vi "hashString.vi"(8 "error in (no error)":errorcluster, 10 "String":string, 11 "HashMap in":refnum<class "HashMap.lvclass">) -> (0 "error out":errorcluster, 2 "Hash":i32, 3 "HashMap out":refnum<class "HashMap.lvclass">)   [LabVIEW 2017, in "HashMap.lvclass"]
uses:
  <userlib>/836-Library/Data_Structures/HashMap/HashMap.lvclass
  <userlib>/836-Library/Data_Structures/HashMap/HashMap.lvclass/HashMap.ctl
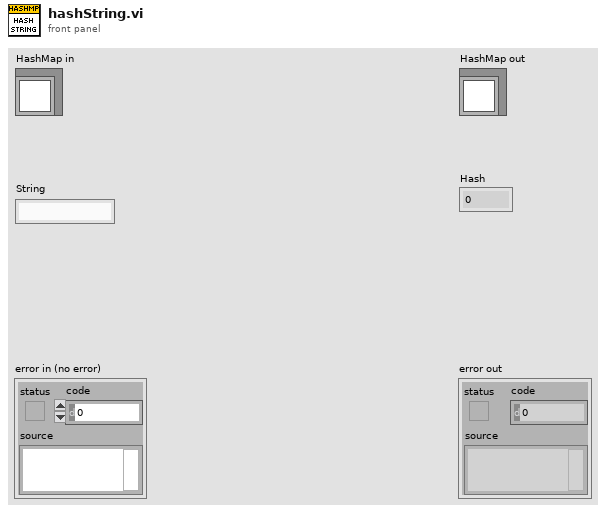
[diagram p1: front panel]
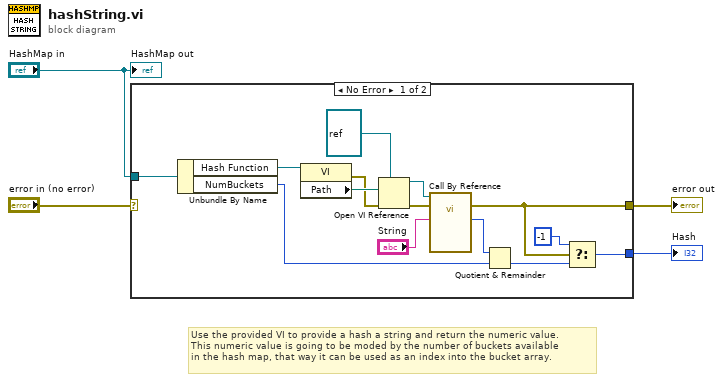
[diagram p0: block diagram]
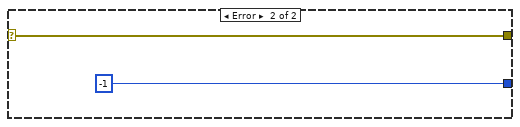
[diagram p2: hidden frame]
diagram:
  # "Use the provided VI to provide a hash a string and return the numeric value.\nThis numeric value is going to be moded by the number of buckets available\nin the hash map, that way it can be used as an index into the bucket array."
  n1 = case shown="No Error" "error in (no error)" {
    selector: "error in (no error)" -> [_ w20]
    tunnel: [w8 w20] -> w3
    tunnel: "HashMap in" -> [w18 _]
    tunnel: [w7 -1] -> w1
    frame No Error {
      n2 = Unbundle By Name(w18) -> ("Hash Function"=w17:refnum<vi>, "NumBuckets"=w9:i32)
      n3 = property class="VI"(reference=w17) -> (error out=w15:errorcluster, "Path"=w16:path)  [unwired: 1 in, 1 out]
      n4 = Open VI Reference(type specifier VI Refnum (for type only)=refnum<vi> refnum, vi path=w16, error in (no error)=w15) -> (vi reference=w13:refnum<vi>, error out=w12:errorcluster)  [unwired: 3 in]
      n5 = call-by-ref "?"(reference=w13, error in=w12, "Key"="String") -> (error out=w8:errorcluster, "Hash"=w10:i32)  [unwired: 10 in, 1 out]
      n6 = Quotient & Remainder(x=w10, y=w9) -> (floor(x/y)=w6:i32)  [unwired: 1 out]
      n7 = Select(t=-1, s=w8, f=w6) -> (s? t:f=w7:i32)
    }
    frame Error {
    }
  }
  "error out" <- w3
  "Hash" <- w1
  "HashMap out" <- "HashMap in"
